vi "SRV_Sensor PARSE_##iL.vi"(0 "Return Data":string) -> (3 "Constant Command":string, 10 "Value":u16)   [LabVIEW 2009]
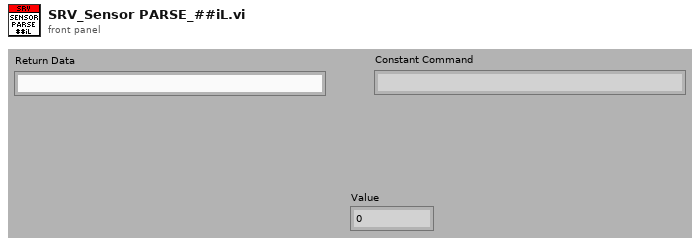
[diagram p1: front panel]
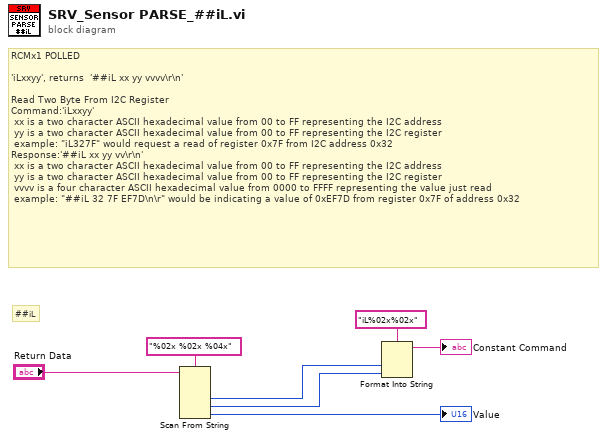
[diagram p0: block diagram]
diagram:
  # "##iL"
  # "RCMx1 POLLED\n\n'iLxxyy', returns  '##iL xx yy vvvv\\r\\n'\n\nRead Two Byte From I2C Register\nCommand:'iLxxyy'\n xx is a two character ASCII hexadecimal value from 00 to FF representing the I2C address\n yy is a two character ASCII hexadecimal value from 00 to FF representing the I2C register\n example: \"iL327F\" would request a read of register 0x7F from I2C address 0x32\nResponse:'##iL xx yy vv\\r\\n'\n xx is a two character ASCII hexadecimal value from 00 to FF representing the I2C address\n yy is a two character ASCII hexadecimal value from 00 to FF representing the I2C register\n vvvv is a four character ASCII hexadecimal value from 0000 to FFFF representing the value just read\n example: \"##iL 32 7F EF7D\\n\\r\" would be indicating a value of 0xEF7D from register 0x7F of address 0x32"
  n1 = Scan From String(format string="%02x %02x %04x", input string="Return Data") -> (output 1=w2:i32, output 2=w1:i32, output 3=→"Value":u16)  [unwired: 5 in, 3 out]
  n2 = Format Into String(format string="iL%02x%02x", w2, w1) -> (resulting string=→"Constant Command":string)  [unwired: 2 in, 1 out]
